vi "FTW-Example-WebSocket-Server-Publisher.vi"() -> ()   [LabVIEW 2015]
panel:
  out "Primary Inbox Address":string="ws://127.0.0.1:65439"
  out "error out":errorcluster
  in  "stop":bool
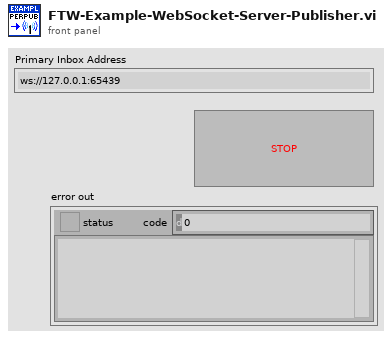
[diagram p1: front panel]
types:
  T1 = typedef "FTW-Type-Socket-Publisher.ctl" = refnum<data-value>
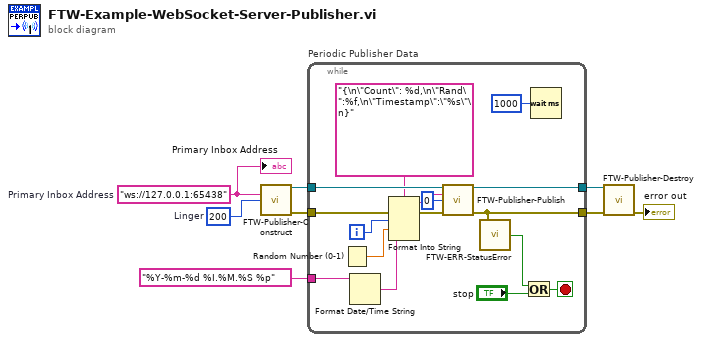
[diagram p0: block diagram]
diagram:
  w6 = 200  # Linger
  w7 = "ws://127.0.0.1:65438"  # Primary Inbox Address
  n1 = call "FTW-Publisher-Construct.vi"("Instance Inbox Address"=w7, "Linger"=w6) -> ("Publisher"=w3:T1, "error out"=w8:errorcluster)  [unwired: 11 in, 1 out]
  n2 = while "Periodic Publisher Data" {
    tunnel: w8 -> [w18]
    tunnel: [w19] -> w4
    tunnel: [w20] -> w2
    tunnel: w3 -> [w21]
    tunnel: "%Y-%m-%d %I.%M.%S %p" ("time format string (%c)") -> [w10]
    i -> [w14]
    stop <- w23 stop-if-true
    n3 = Random Number (0-1)() -> (number: 0 to 1=w13:dbl)
    n4 = Format Date/Time String(time format string (%c)=w10) -> (date/time string=w11:string)  [unwired: 2 in]
    n5 = Format Into String(format string="{\n\"Count\": %d,\n\"Rand\":%f,\n\"Timestamp\":\"%s\"\n}" ("Message"), error in=w18, w14, w13, w11) -> (resulting string=w16:string, error out=w17:errorcluster)  [unwired: 1 in]
    n6 = call "FTW-Publisher-Publish.vi"("Publisher"=w21, "Message"=w16, "Send Timeout"=0, "error in"=w17) -> ("Publisher out"=w20:T1, "error out"=w19:errorcluster)  [unwired: 10 in]
    n7 = call "FTW-ERR-StatusError.vi"("error to check"=w19) -> ("Error?"=w24:bool)
    n8 = Or(x=w24, y="stop") -> (x .or. y?=w23:bool)
    n9 = Wait (ms)(milliseconds to wait=u32 1000) -> ()  [unwired: 1 out]
  }
  n10 = call "FTW-Publisher-Destroy.vi"("Publisher"=w2, "error in"=w4) -> ("error out"=→"error out":errorcluster)  [unwired: 13 in]
  "Primary Inbox Address" <- w7
